vi "Generate3DTrain.vi"(8 "error in":errorcluster, 11 "Local":T6={"Parameter"={"3D Plot"=[], "3D Scatter"=refnum, "Data"={"Split"={"X Train"=[], "X Test"=[], "Y Train"=[], "Y Test"=[]}, "Predict"=[]}, "Display"={"Choice"=enum."All", "Indexe"={"X"=0, "Y"=1, "Z"=2}}, "Point Property"={"Train Style"=enum."Full circle", "Test OK Style"=enum."Full square", "Label Color"=[8978528, 4367871, 1985280], "Test NO OK"={"Style"=enum."Cross", "Color"=16716800}}, "3D Plot Datatype.lvclass"=refnum}, "3DArray"=[], "Rating 3D Array"=[], "GoodPredict"=0, "Point ID"=[]}) -> (0 "error out":errorcluster, 3 "Local Out":T6={"Parameter"={"3D Plot"=[], "3D Scatter"=refnum, "Data"={"Split"={"X Train"=[], "X Test"=[], "Y Train"=[], "Y Test"=[]}, "Predict"=[]}, "Display"={"Choice"=enum."All", "Indexe"={"X"=0, "Y"=0, "Z"=2}}, "Point Property"={"Train Style"=enum."Empty circle", "Test OK Style"=enum."Empty circle", "Label Color"=[], "Test NO OK"={"Style"=enum."Empty circle", "Color"=0}}, "3D Plot Datatype.lvclass"=refnum}, "3DArray"=[], "Rating 3D Array"=[], "GoodPredict"=0, "Point ID"=[]})   [LabVIEW 2020]
doc: "Generate 3D array"
uses:
  _Controls/3DParameters.ctl
  <vilib>/Math Plots/3D Math Plots/3D Plot/3D Plot Datatype/3D Plot Datatype.lvclass
  <vilib>/Math Plots/3D Math Plots/3D Scatter/3D Scatter XCtrl/3D Scatter.xctl
  _Controls/Datas.ctl
  _Controls/PointPropertyMultipleLabel.ctl
  _Controls/Style.ctl
  _Controls/3DData.ctl
types:
  T1 = typedef "3DParameters.ctl" = cluster{"3D Plot":refnum<class "3D Plot Datatype.lvclass">[], "3D Scatter":refnum<vi>, "Data":T2, "Display":cluster{"Choice":enum16{"All", "Train", "Test"}, "Indexe":cluster{"X":i32, "Y":i32, "Z":i32}}, "Point Property":T3, "3D Plot Datatype.lvclass":refnum<class "3D Plot Datatype.lvclass">}
  T2 = typedef "Datas.ctl" = cluster{"Split":cluster{"X Train":dbl[][], "X Test":dbl[][], "Y Train":dbl[][], "Y Test":dbl[][]}, "Predict":dbl[][]}
  T3 = typedef "PointPropertyMultipleLabel.ctl" = cluster{"Train Style":T4, "Test OK Style":T4, "Label Color":u32[], "Test NO OK":cluster{"Style":T4, "Color":u32}}
  T4 = typedef "Style.ctl" = enum16{"Empty circle", "Full circle", "Empty square", "Full square", "Cross"}
  T5 = typedef "3DData.ctl" = cluster{"Tag":i32, "X":dbl[], "Y":dbl[], "Z":dbl[]}
  T6 = cluster{"Parameter":T1, "3DArray":cluster{"X":dbl[], "Y":dbl[], "Z":dbl[]}[], "Rating 3D Array":T5[], "GoodPredict":i32, "Point ID":cluster{"DataUse":enum16{"Dataset", "Train", "Test"}, "Color":u32}[]}
  T7 = cluster{"DataUse":enum16{"Dataset", "Train", "Test"}, "Color":u32}
  T8 = cluster{"X Train":dbl[][], "X Test":dbl[][], "Y Train":dbl[][], "Y Test":dbl[][]}
  T9 = cluster{"DataUse":enum16{"Dataset", "Train", "Test"}, "Color":u32}[]
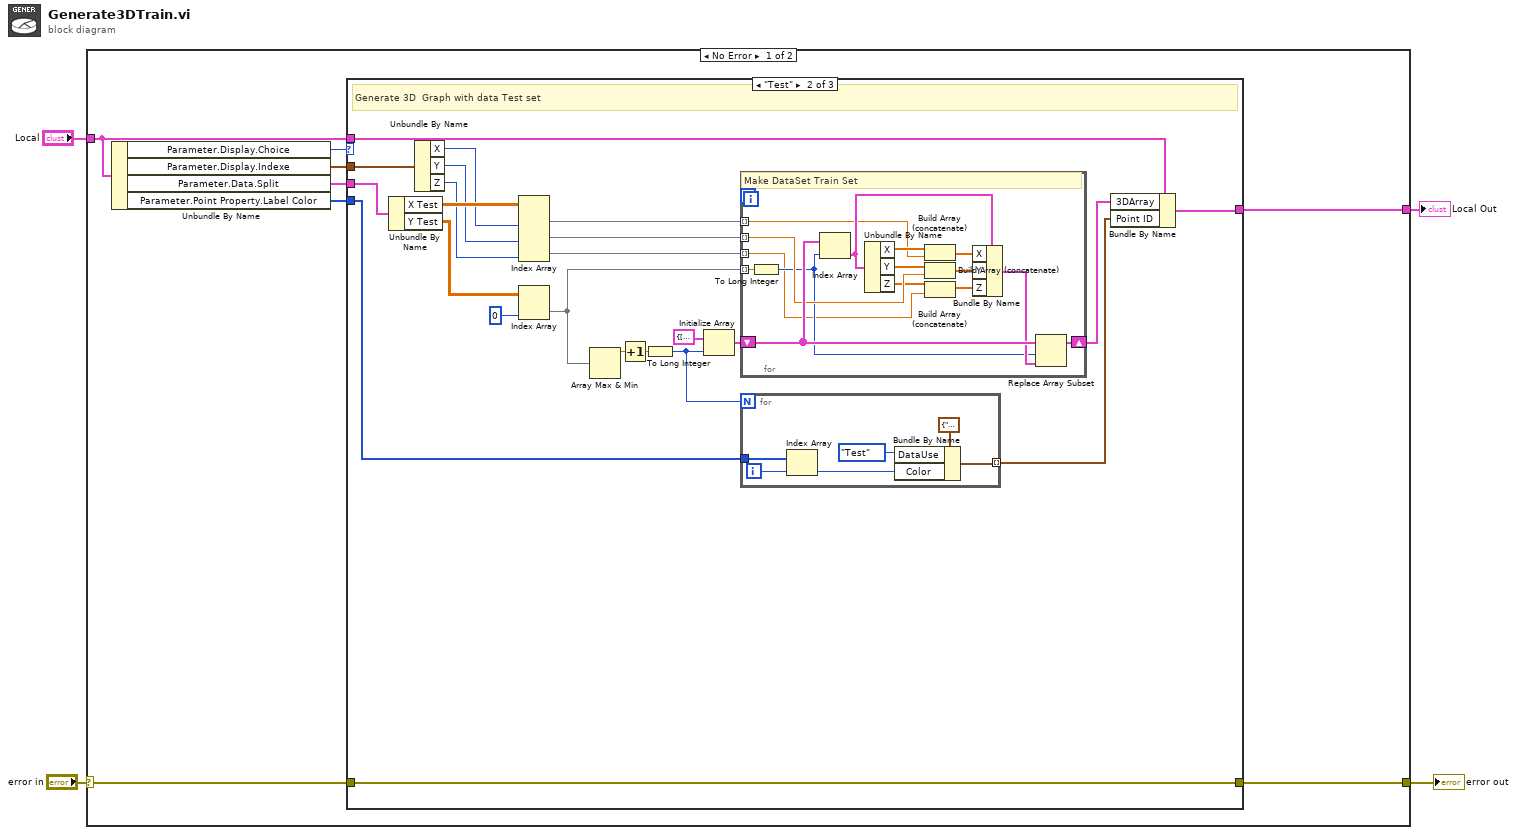
[diagram p0: block diagram]
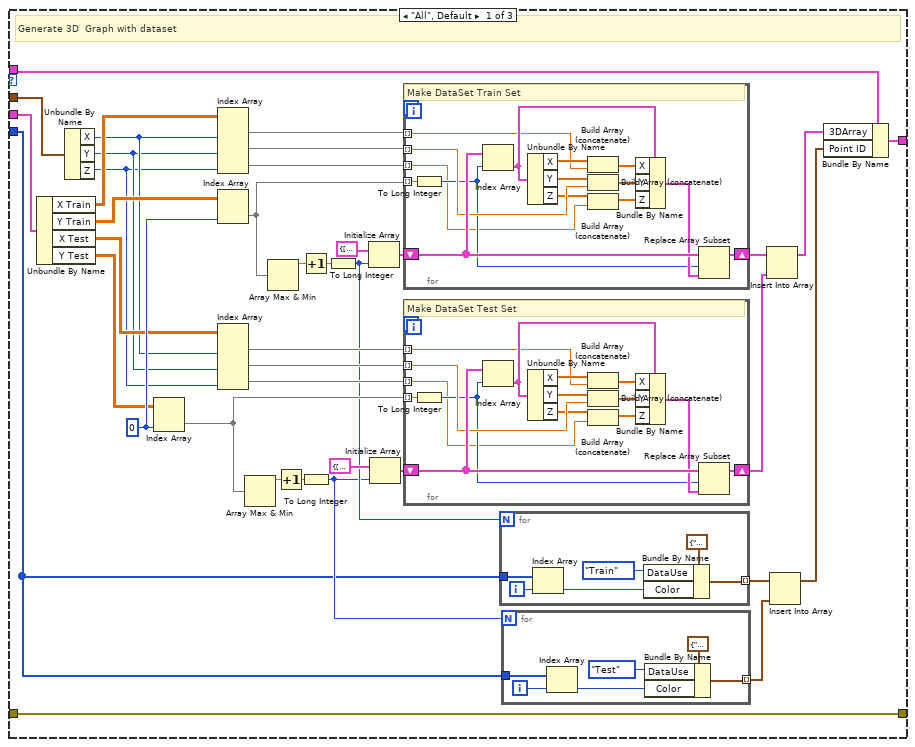
[diagram p2: hidden frame]
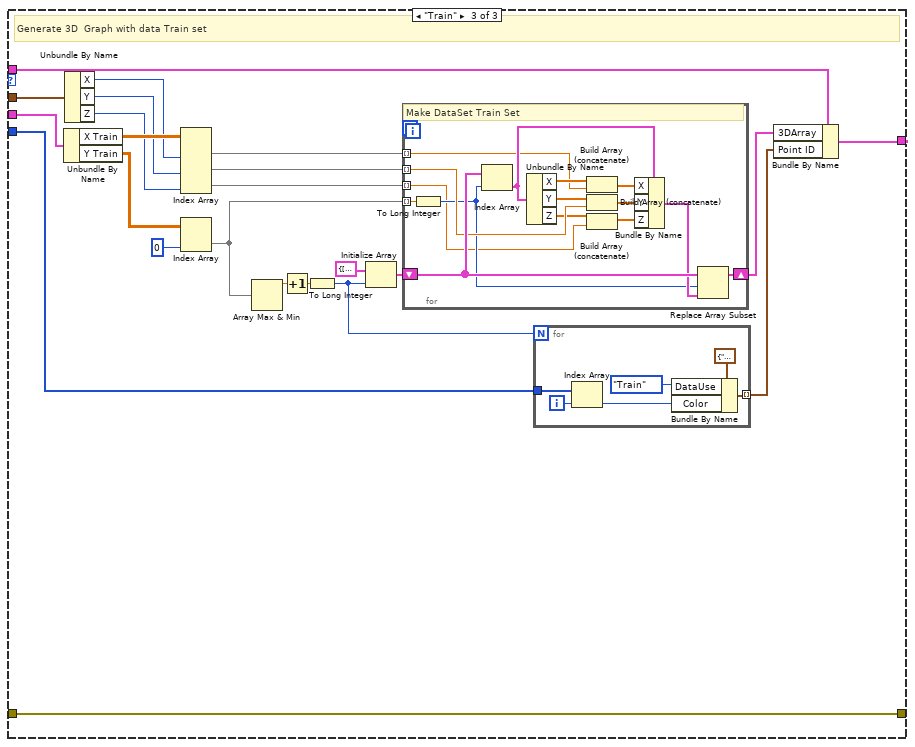
[diagram p3: hidden frame]
diagram:
  n1 = case shown="No Error" "error in" {
    selector: "error in" -> [w10 w181]
    tunnel: "Local" -> [w11 w182]
    tunnel: [w9 w182] -> w1
    tunnel: [w8 w181] -> w3
    frame No Error {
      n2 = Unbundle By Name(w11) -> ("Parameter.Display.Choice"=w12:enum16{"All", "Train", "Test"}, "Parameter.Display.Indexe"=w7:cluster{"X":i32, "Y":i32, "Z":i32}, "Parameter.Data.Split"=w6:T8, "Parameter.Point Property.Label Color"=w5:u32[])
      n3 = case shown="\"Test\"" w12 {
        tunnel: w10 -> [w17 w97 w140]
        tunnel: w11 -> [w14 w96 w141]
        tunnel: [w50 w108 w152] -> w9
        tunnel: [w17 w97 w140] -> w8
        tunnel: w7 -> [w15 w95 w139]
        tunnel: w6 -> [w16 w94 w138]
        tunnel: w5 -> [w13 w93 w137]
        frame "All", Default {
          w28 = 0 ("index (col)")
          # "Generate 3D  Graph with dataset"
          n4 = Unbundle By Name(w16) -> ("X Train"=w27:dbl[][], "Y Train"=w26:dbl[][], "X Test"=w25:dbl[][], "Y Test"=w21:dbl[][])
          n5 = Unbundle By Name(w15) -> ("X"=w24:i32, "Y"=w23:i32, "Z"=w22:i32)
          n6 = Index Array(array=w21, index (col)=w28) -> (element=w40:dbl[])  [unwired: 1 in]
          n7 = Index Array(array=w27, index (col) #1=w24, index (col) #2=w23, index (col) #3=w22) -> (element #1=w38:dbl[], element #2=w37:dbl[], element #3=w36:dbl[])  [unwired: 3 in]
          n8 = Index Array(array=w26, index (col)=w28) -> (element=w32:dbl[])  [unwired: 1 in]
          n9 = Index Array(array=w25, index (col) #1=w24, index (col) #2=w23, index (col) #3=w22) -> (element #1=w44:dbl[], element #2=w45:dbl[], element #3=w39:dbl[])  [unwired: 3 in]
          n10 = Array Max & Min(array=w40) -> (max value=w42:dbl)  [unwired: 3 out]
          n11 = Array Max & Min(array=w32) -> (max value=w34:dbl)  [unwired: 3 out]
          n12 = Increment(x=w42) -> (x+1=w46:dbl)
          n13 = Increment(x=w34) -> (x+1=w33:dbl)
          n14 = To Long Integer(number=w46) -> (32bit integer=w19:i32)
          n15 = To Long Integer(number=w33) -> (32bit integer=w20:i32)
          n16 = Initialize Array(cluster{"X":dbl[], "Y":dbl[], "Z":dbl[]} {"X"=[], "Y"=[], "Z"=[]} ("Cluster"), w20) -> (w31:cluster{"X":dbl[], "Y":dbl[], "Z":dbl[]}[])
          n17 = Initialize Array(cluster{"X":dbl[], "Y":dbl[], "Z":dbl[]} {"X"=[], "Y"=[], "Z"=[]} ("Cluster"), w19) -> (w43:cluster{"X":dbl[], "Y":dbl[], "Z":dbl[]}[])
          n18 = for {
            tunnel: w37 -> [w57] mode=indexing
            tunnel: w38 -> [w55] mode=indexing
            tunnel: w32 -> [w59] mode=indexing
            shift-right: [w61] -> w30
            shift-left: w31 -> [w62]
            tunnel: w36 -> [w52] mode=indexing
            # "Make DataSet Train Set"
            n19 = To Long Integer(number=w59) -> (32bit integer=w54:i32)
            n20 = Index Array(array=w62, index=w54) -> (element=w65:cluster{"X":dbl[], "Y":dbl[], "Z":dbl[]})
            n21 = Unbundle By Name(w65) -> ("X"=w56:dbl[], "Y"=w58:dbl[], "Z"=w53:dbl[])
            n22 = Build Array (concatenate)(w56, w55) -> (w64:dbl[])
            n23 = Build Array (concatenate)(w58, w57) -> (w63:dbl[])
            n24 = Build Array (concatenate)(w53, w52) -> (w51:dbl[])
            n25 = Bundle By Name(cluster=w65, "X"=w64, "Y"=w63, "Z"=w51) -> (w60:cluster{"X":dbl[], "Y":dbl[], "Z":dbl[]})
            n26 = Replace Array Subset(array=w62, new element=w60, index=w54) -> (w61:cluster{"X":dbl[], "Y":dbl[], "Z":dbl[]}[])
          }
          n27 = for {
            tunnel: w45 -> [w72] mode=indexing
            tunnel: w44 -> [w70] mode=indexing
            tunnel: w40 -> [w74] mode=indexing
            shift-right: [w76] -> w29
            shift-left: w43 -> [w77]
            tunnel: w39 -> [w67] mode=indexing
            # "Make DataSet Test Set"
            n28 = To Long Integer(number=w74) -> (32bit integer=w69:i32)
            n29 = Index Array(array=w77, index=w69) -> (element=w80:cluster{"X":dbl[], "Y":dbl[], "Z":dbl[]})
            n30 = Unbundle By Name(w80) -> ("X"=w71:dbl[], "Y"=w73:dbl[], "Z"=w68:dbl[])
            n31 = Build Array (concatenate)(w71, w70) -> (w79:dbl[])
            n32 = Build Array (concatenate)(w73, w72) -> (w78:dbl[])
            n33 = Build Array (concatenate)(w68, w67) -> (w66:dbl[])
            n34 = Bundle By Name(cluster=w80, "X"=w79, "Y"=w78, "Z"=w66) -> (w75:cluster{"X":dbl[], "Y":dbl[], "Z":dbl[]})
            n35 = Replace Array Subset(array=w77, new element=w75, index=w69) -> (w76:cluster{"X":dbl[], "Y":dbl[], "Z":dbl[]}[])
          }
          n36 = for {
            N: w20 -> [_]
            tunnel: [w92] -> w49 mode=indexing
            tunnel: w13 -> [w87]
            i -> [w89]
            n37 = Index Array(array=w87, index=w89) -> (element=w88:u32)
            n38 = Bundle By Name(cluster=T7 {"DataUse"=enum."Train", "Color"=0}, "DataUse"=enum16{"Dataset", "Train", "Test"}."Train", "Color"=w88) -> (w92:T7)
          }
          n39 = for {
            N: w19 -> [_]
            tunnel: [w86] -> w48 mode=indexing
            tunnel: w13 -> [w81]
            i -> [w83]
            n40 = Index Array(array=w81, index=w83) -> (element=w82:u32)
            n41 = Bundle By Name(cluster=T7 {"DataUse"=enum."Train", "Color"=0}, "DataUse"=enum16{"Dataset", "Train", "Test"}."Test", "Color"=w82) -> (w86:T7)
          }
          n42 = Insert Into Array(array=w30, new element=w29) -> (w18:cluster{"X":dbl[], "Y":dbl[], "Z":dbl[]}[])  [unwired: 1 in]
          n43 = Insert Into Array(array=w49, new element=w48) -> (w47:T9)  [unwired: 1 in]
          n44 = Bundle By Name(cluster=w14, "3DArray"=w18, "Point ID"=w47) -> (w50:T6)
        }
        frame "Test" {
          # "Generate 3D  Graph with data Test set"
          n45 = Unbundle By Name(w94) -> ("X Test"=w112:dbl[][], "Y Test"=w111:dbl[][])
          n46 = Unbundle By Name(w95) -> ("X"=w109:i32, "Y"=w110:i32, "Z"=w103:i32)
          n47 = Index Array(array=w112, index (col) #1=w109, index (col) #2=w110, index (col) #3=w103) -> (element #1=w106:dbl[], element #2=w105:dbl[], element #3=w102:dbl[])  [unwired: 3 in]
          n48 = Index Array(array=w111, index (col)=0 ("index of element")) -> (element=w104:dbl[])  [unwired: 1 in]
          n49 = Array Max & Min(array=w104) -> (max value=w114:dbl)  [unwired: 3 out]
          n50 = Increment(x=w114) -> (x+1=w115:dbl)
          n51 = To Long Integer(number=w115) -> (32bit integer=w98:i32)
          n52 = Initialize Array(cluster{"X":dbl[], "Y":dbl[], "Z":dbl[]} {"X"=[], "Y"=[], "Z"=[]} ("Cluster"), w98) -> (w101:cluster{"X":dbl[], "Y":dbl[], "Z":dbl[]}[])
          n53 = for {
            tunnel: w105 -> [w122] mode=indexing
            tunnel: w106 -> [w120] mode=indexing
            tunnel: w104 -> [w124] mode=indexing
            shift-right: [w126] -> w99
            shift-left: w101 -> [w127]
            tunnel: w102 -> [w117] mode=indexing
            # "Make DataSet Train Set"
            n54 = To Long Integer(number=w124) -> (32bit integer=w119:i32)
            n55 = Index Array(array=w127, index=w119) -> (element=w130:cluster{"X":dbl[], "Y":dbl[], "Z":dbl[]})
            n56 = Unbundle By Name(w130) -> ("X"=w121:dbl[], "Y"=w123:dbl[], "Z"=w118:dbl[])
            n57 = Build Array (concatenate)(w121, w120) -> (w129:dbl[])
            n58 = Build Array (concatenate)(w123, w122) -> (w128:dbl[])
            n59 = Build Array (concatenate)(w118, w117) -> (w116:dbl[])
            n60 = Bundle By Name(cluster=w130, "X"=w129, "Y"=w128, "Z"=w116) -> (w125:cluster{"X":dbl[], "Y":dbl[], "Z":dbl[]})
            n61 = Replace Array Subset(array=w127, new element=w125, index=w119) -> (w126:cluster{"X":dbl[], "Y":dbl[], "Z":dbl[]}[])
          }
          n62 = for {
            N: w98 -> [_]
            tunnel: [w136] -> w107 mode=indexing
            tunnel: w93 -> [w131]
            i -> [w133]
            n63 = Index Array(array=w131, index=w133) -> (element=w132:u32)
            n64 = Bundle By Name(cluster=T7 {"DataUse"=enum."Train", "Color"=0}, "DataUse"=enum16{"Dataset", "Train", "Test"}."Test", "Color"=w132) -> (w136:T7)
          }
          n65 = Bundle By Name(cluster=w96, "3DArray"=w99, "Point ID"=w107) -> (w108:T6)
        }
        frame "Train" {
          # "Generate 3D  Graph with data Train set"
          n66 = Unbundle By Name(w138) -> ("X Train"=w156:dbl[][], "Y Train"=w155:dbl[][])
          n67 = Unbundle By Name(w139) -> ("X"=w153:i32, "Y"=w154:i32, "Z"=w148:i32)
          n68 = Index Array(array=w156, index (col) #1=w153, index (col) #2=w154, index (col) #3=w148) -> (element #1=w151:dbl[], element #2=w150:dbl[], element #3=w147:dbl[])  [unwired: 3 in]
          n69 = Index Array(array=w155, index (col)=0 ("index of element")) -> (element=w149:dbl[])  [unwired: 1 in]
          n70 = Array Max & Min(array=w149) -> (max value=w158:dbl)  [unwired: 3 out]
          n71 = Increment(x=w158) -> (x+1=w159:dbl)
          n72 = To Long Integer(number=w159) -> (32bit integer=w144:i32)
          n73 = Initialize Array(cluster{"X":dbl[], "Y":dbl[], "Z":dbl[]} {"X"=[], "Y"=[], "Z"=[]} ("Cluster"), w144) -> (w146:cluster{"X":dbl[], "Y":dbl[], "Z":dbl[]}[])
          n74 = for {
            tunnel: w150 -> [w166] mode=indexing
            tunnel: w151 -> [w164] mode=indexing
            tunnel: w149 -> [w168] mode=indexing
            shift-right: [w170] -> w143
            shift-left: w146 -> [w171]
            tunnel: w147 -> [w161] mode=indexing
            # "Make DataSet Train Set"
            n75 = To Long Integer(number=w168) -> (32bit integer=w163:i32)
            n76 = Index Array(array=w171, index=w163) -> (element=w174:cluster{"X":dbl[], "Y":dbl[], "Z":dbl[]})
            n77 = Unbundle By Name(w174) -> ("X"=w165:dbl[], "Y"=w167:dbl[], "Z"=w162:dbl[])
            n78 = Build Array (concatenate)(w165, w164) -> (w173:dbl[])
            n79 = Build Array (concatenate)(w167, w166) -> (w172:dbl[])
            n80 = Build Array (concatenate)(w162, w161) -> (w160:dbl[])
            n81 = Bundle By Name(cluster=w174, "X"=w173, "Y"=w172, "Z"=w160) -> (w169:cluster{"X":dbl[], "Y":dbl[], "Z":dbl[]})
            n82 = Replace Array Subset(array=w171, new element=w169, index=w163) -> (w170:cluster{"X":dbl[], "Y":dbl[], "Z":dbl[]}[])
          }
          n83 = for {
            N: w144 -> [_]
            tunnel: [w180] -> w142 mode=indexing
            tunnel: w137 -> [w175]
            i -> [w177]
            n84 = Index Array(array=w175, index=w177) -> (element=w176:u32)
            n85 = Bundle By Name(cluster=T7 {"DataUse"=enum."Train", "Color"=0}, "DataUse"=enum16{"Dataset", "Train", "Test"}."Train", "Color"=w176) -> (w180:T7)
          }
          n86 = Bundle By Name(cluster=w141, "3DArray"=w143, "Point ID"=w142) -> (w152:T6)
        }
      }
    }
    frame Error {
    }
  }
  "error out" <- w3
  "Local Out" <- w1
